vi "Window-Funct TIFF export.vi"() -> ()   [LabVIEW 2020]
uses:
  Processing/Patches/Typedefs/Functional TIFF exporter states.ctl
  System.Windows.Forms
  Processing/Patches/Typedefs/Exported TIFF type.ctl
  Processing/Patches/Typedefs/Funct TIFF exporter ctrl refs.ctl
  <vilib>/Utility/miscctls.llb/LVPointTypeDef.ctl
  Processing/Patches/Globals/gl_funct TIFF export globals.vi
  Global Variables/General Globals.vi
panel:
  out "Experiment Header":string
  in  "Output tupe":T1
  out "Trial number":string
  out "Close":bool
  out "Predominant ROI type":string="Predominant ROI type:"
  out "Imaging protocol":string="Imaging protocol:"
  out "State":T2
  in  "Export":bool
  out "Current Experiment":string="Current experiment:"
  out "Patches in Experiment":i32 format="%.0f Patches in this experiment"
  in  "Folder Path":path
  in  "ProgressBar":refnum<k24>(container)
  # "This utility exports individual rectangles from functional imaging's raw data"
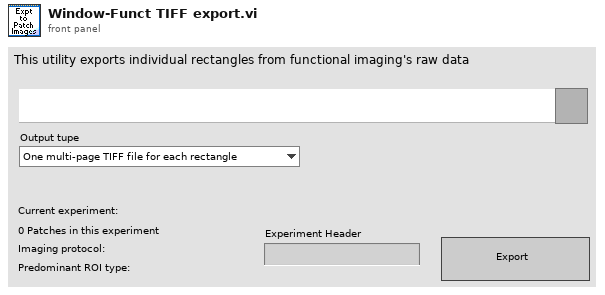
[diagram p1: front panel]
types:
  T1 = typedef "Exported TIFF type.ctl" = enum16{"One multi-page TIFF file for each rectangle", "Individual TIFF files"}
  T2 = typedef "Functional TIFF exporter states.ctl" = enum16{"Idle", "Export"}
  T3 = typedef "Funct TIFF exporter ctrl refs.ctl" = cluster{"This VI":refnum<vi>, "Current Experiment":refnum<vi>, "Imaging protocol":refnum<vi>, "Predominant ROI type":refnum<vi>, "Patches in Experiment":refnum<vi>, "Folder Path":refnum<vi>, "Export":refnum<vi>, "Trial number":refnum<vi>, "Output TIFF type":refnum<vi>}
  T4 = typedef "LVPointTypeDef.ctl" = cluster{"Horizontal":i16, "Vertical":i16}
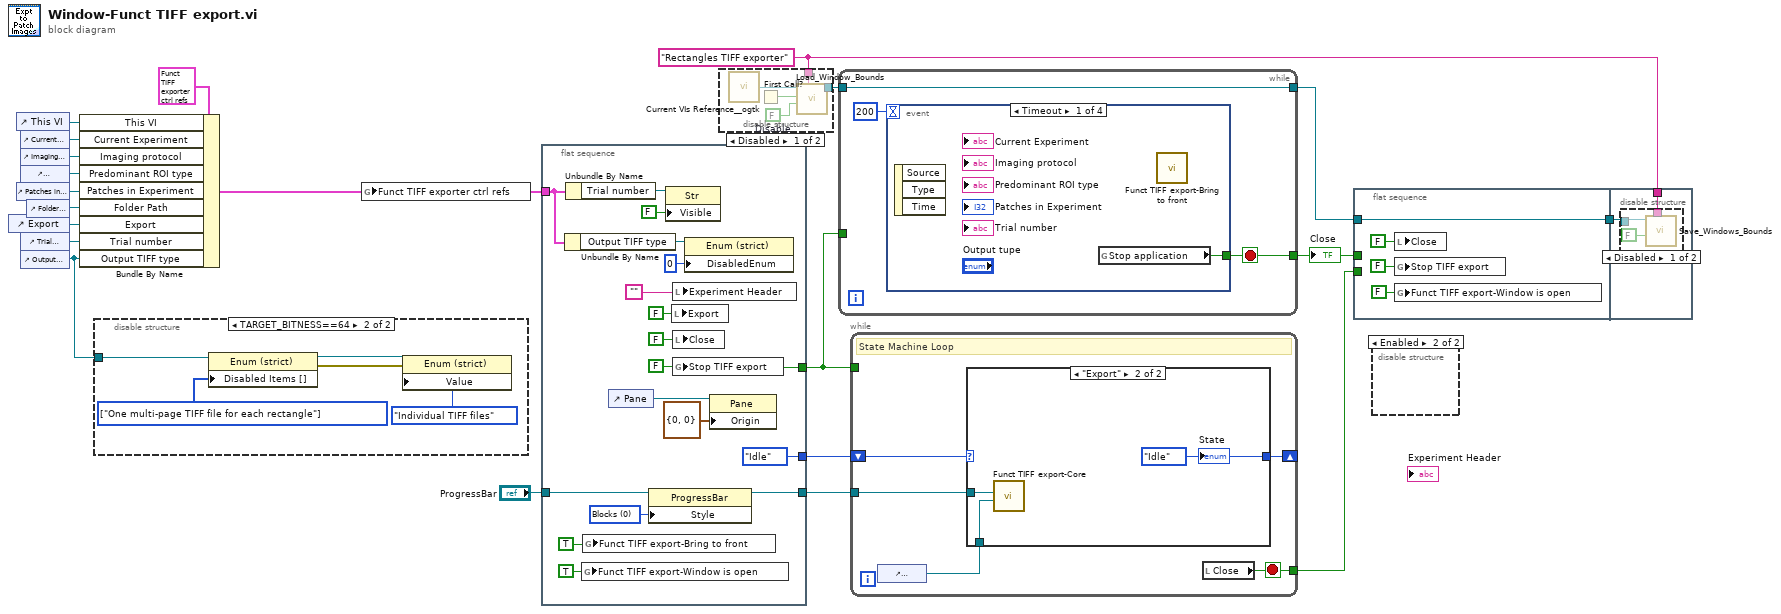
[diagram p0: block diagram]
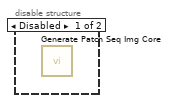
[diagram p4: hidden frame]
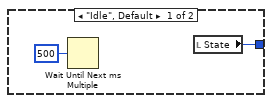
[diagram p6: hidden frame]
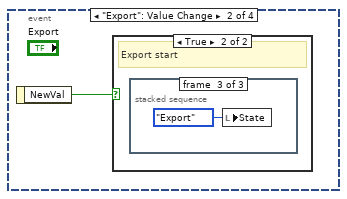
[diagram p7: hidden frame]
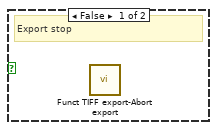
[diagram p8: hidden frame]
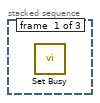
[diagram p9: hidden frame]
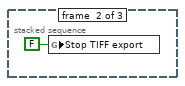
[diagram p10: hidden frame]
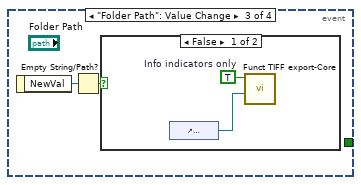
[diagram p11: hidden frame]
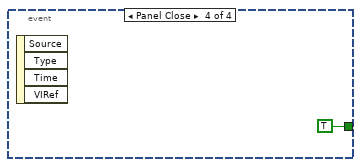
[diagram p13: hidden frame]
diagram:
  w10 = "Rectangles TIFF exporter" ("Window Name (i.e. Key)")
  n1 = control-ref of="Export"() -> (w3:refnum<vi>)
  n2 = control-ref of="This VI"() -> (w7:refnum<vi>)
  n3 = control-ref of="Patches in Experiment"() -> (w13:refnum<vi>)
  n4 = control-ref of="Current Experiment"() -> (w17:refnum<vi>)
  n5 = control-ref of="Imaging protocol"() -> (w16:refnum<vi>)
  n6 = control-ref of="Predominant ROI type"() -> (w15:refnum<vi>)
  n7 = control-ref of="Trial number"() -> (w2:refnum<vi>)
  n8 = control-ref of="Output tupe"() -> (w1:refnum<vi>)
  n9 = control-ref of="Folder Path"() -> (w11:refnum<vi>)
  n10 = Bundle By Name(cluster=T3 {"This VI"=refnum, "Current Experiment"=refnum, "Imaging protocol"=refnum, "Predominant ROI type"=refnum, "Patches in Experiment"=refnum, "Folder Path"=refnum, "Export"=refnum, "Trial number"=refnum, "Output TIFF type"=refnum} ("output cluster"), "This VI"=w7, "Current Experiment"=w17, "Imaging protocol"=w16, "Predominant ROI type"=w15, "Patches in Experiment"=w13, "Folder Path"=w11, "Export"=w3, "Trial number"=w2, "Output TIFF type"=w1) -> (w12:T3)
  n11 = disable-structure shown="TARGET_BITNESS==64" {
    disable-tunnel: w1 -> [_ w22]
    frame condition #0 {
    }
    frame condition #1 (active) {
      w26 = T1[] [enum."One multi-page TIFF file for each rectangle"] items=["One multi-page TIFF file for each rectangle", "Individual TIFF files"]
      n12 = property class="Enum (strict)"(reference=w22, "Disabled Items []"=w26) -> (reference out=w24:refnum<vi>, error out=w25:errorcluster)  [unwired: 1 in]
      n13 = property class="Enum (strict)"(reference=w24, error in=w25, "Value"=Exported_TIFF_type."Individual TIFF files") -> ()  [unwired: 2 out]
    }
  }
  n14 = global write "gl_funct TIFF export globals.vi" "Funct TIFF exporter ctrl refs"(w12) -> ()
  n15 = flat-sequence {
    tunnel: [w43] -> w18
    tunnel: w12 -> [w28]
    tunnel: "ProgressBar" -> [w35]
    tunnel: [Functional_TIFF_exporter_states."Idle" ("State")] -> w6
    tunnel: [w33] -> w5
    frame #0 {
      w36 = 0 items=["Blocks", "Continuous", "Marquee"] ("Style")
      w43 = FALSE ("Stop TIFF export")
      n16 = Unbundle By Name(w28) -> ("Output TIFF type"=w30:refnum<vi>)
      n17 = Unbundle By Name(w28) -> ("Trial number"=w32:refnum<vi>)
      n18 = global write "gl_funct TIFF export globals.vi" "Funct TIFF export-Window is open"(TRUE ("Funct TIFF export-Window is open")) -> ()
      n19 = global write "gl_funct TIFF export globals.vi" "Funct TIFF export-Bring to front"(TRUE ("Bring Timelapse Editor to front")) -> ()
      n20 = control-ref of="Pane"() -> (w42:refnum<vi>)
      n21 = property class="ProgressBar"(reference=w35, "Style"=w36) -> (reference out=w33:refnum<k24>)  [unwired: 1 in, 1 out]
      n22 = property class="Str"(reference=w32, "Visible"=FALSE) -> ()  [unwired: 1 in, 2 out]
      n23 = local write "Export"(FALSE ("Export")) -> ()
      n24 = local write "Experiment Header"("") -> ()
      n25 = local write "Close"(FALSE ("Close")) -> ()
      n26 = global write "gl_funct TIFF export globals.vi" "Stop TIFF export"(w43) -> ()
      n27 = property class="Enum (strict)"(reference=w30, "DisabledEnum"=0) -> ()  [unwired: 1 in, 2 out]
      n28 = property class="Pane"(reference=w42, "Origin"=T4 {"Horizontal"=0, "Vertical"=0}) -> ()  [unwired: 1 in, 2 out]
    }
  }
  n29 = disable-structure shown="Disabled" {
    disable-tunnel: [w48 _] -> w21
    disable-tunnel: w10 -> [w47 _]
    frame Disabled {
      w45 = FALSE  # Disable
      n30 = call <userlib>:"Current VIs Reference__ogtk.vi"() -> ("Current VI's reference"=w46:refnum<vi>)  [unwired: 5 in]
      n31 = First Call?() -> (First Call?: T/F=w44:bool)
      n32 = call "Load_Window_Bounds.vi"("Window Name (i.e. Key)"=w47, "Disable"=w45, "First Call"=w44, "Window VI's Ref"=w46) -> ("reference out"=w48:refnum<vi>)  [unwired: 4 in, 3 out]
    }
    frame Enabled {
    }
  }
  n33 = while {
    tunnel: w21 -> [w50]
    tunnel: [w50] -> w8
    tunnel: [w49] -> w20
    tunnel: w18 -> [_]
    stop <- w49 stop-if-true
    n34 = event shown="[0] Timeout" {
      selector: _ -> [_ _ _ _]
      dyn-events: _ -> [_ _ _ _]
      timeout: 200 -> [_ _ _ _]
      tunnel: [w52 _ _ TRUE] -> w49
      event Timeout {
        n35 = event-data() -> ()  [unwired: 1 in, 3 out]
        n36 = global read "General Globals.vi" "Stop application"() -> (w52:bool)
        n37 = call "Funct TIFF export-Bring to front.vi"() -> ()  [unwired: 12 in]
      }
      event "Export": Value Change {
        n38 = event-data() -> ("NewVal"=w53:bool)  [unwired: 1 in]
        n39 = case shown="True" w53 {
          frame False {
            # "Export stop"
            n40 = call "Funct TIFF export-Abort export.vi"() -> ()  [unwired: 12 in]
          }
          frame True {
            # "Export start"
            n41 = stacked-sequence {
              frame #0 {
                n42 = call <vilib>:"Set Busy.vi"() -> ()  [unwired: 10 in, 2 out]
              }
              frame #1 {
                n43 = global write "gl_funct TIFF export globals.vi" "Stop TIFF export"(FALSE ("Stop TIFF export")) -> ()
              }
              frame #2 {
                n44 = local write "State"(Functional_TIFF_exporter_states."Export" ("State")) -> ()
              }
            }
          }
        }
      }
      event "Folder Path": Value Change {
        n45 = event-data() -> ("NewVal"=w56:path)  [unwired: 1 in]
        n46 = Empty String/Path?(string/path=w56) -> (empty?=w57:bool)
        n47 = case shown="False" w57 {
          frame False {
            w59 = TRUE  # Info indicators only
            n48 = control-ref of="Experiment Header"() -> (w58:refnum<vi>)
            n49 = call "Funct TIFF export-Core.vi"("Experiment Header string"=w58, "Info indicators only (F)"=w59) -> ()  [unwired: 10 in]
          }
          frame True {
          }
        }
      }
      event Panel Close {
        n50 = event-data() -> ()  [unwired: 1 in, 4 out]
      }
    }
  }
  "Close" <- w20
  n51 = while {
    shift-right: [w64] -> _
    shift-left: w6 -> [w65]
    tunnel: [w63] -> w19
    tunnel: w18 -> [_]
    tunnel: w5 -> [w62]
    stop <- w63 stop-if-true
    # "State Machine Loop"
    n52 = control-ref of="Experiment Header"() -> (w61:refnum<vi>)
    n53 = case shown="\"Export\"" w65 {
      tunnel: [w66 w70] -> w64
      tunnel: w62 -> [_ w69]
      tunnel: w61 -> [_ w68]
      frame "Idle", Default {
        n54 = Wait Until Next ms Multiple(millisecond multiple=u32 500) -> ()  [unwired: 1 out]
        n55 = local read "State"() -> (w66:T2)
      }
      frame "Export" {
        w70 = Functional_TIFF_exporter_states."Idle" ("State")
        n56 = call "Funct TIFF export-Core.vi"("Experiment Header string"=w68, "ProgressBar"=w69) -> ()  [unwired: 10 in]
        "State" <- w70
      }
    }
    n57 = local read "Close"() -> (w63:bool)
  }
  n58 = flat-sequence {
    tunnel: w20 -> [_]
    tunnel: w19 -> [_]
    tunnel: [w72] -> w9
    tunnel: w8 -> [w72]
    tunnel: w10 -> [w76]
    tunnel: w9 -> [w75]
    frame #0 {
      n59 = local write "Close"(FALSE ("Close")) -> ()
      n60 = global write "gl_funct TIFF export globals.vi" "Stop TIFF export"(FALSE ("Stop TIFF export")) -> ()
      n61 = global write "gl_funct TIFF export globals.vi" "Funct TIFF export-Window is open"(FALSE ("Funct TIFF export-Window is open")) -> ()
    }
    frame #1 {
      n62 = disable-structure shown="Disabled" {
        disable-tunnel: w76 -> [w79 _]
        disable-tunnel: w75 -> [w78 _]
        frame Disabled {
          n63 = call "Save_Windows_Bounds.vi"("Window Name (i.e. Key)"=w79, "Front Panel Window:Open"=FALSE, "Window VI's Ref"=w78) -> ()  [unwired: 8 in, 1 out]
        }
        frame Enabled {
        }
      }
    }
  }
  n64 = disable-structure shown="Enabled" {
    frame Disabled {
      n65 = call "Generate Patch Seq Img Core.vi"() -> ()  [unwired: 14 in, 2 out]
    }
    frame Enabled {
    }
  }
